vi "get_settings_cluster.vi"(8 "error in (no error)":errorcluster, 11 "GenericPlugin in":refnum<class "StimulatorDL090503.lvclass">) -> (0 "error out":errorcluster, 2 "settings cluster":variant, 3 "GenericPlugin out":refnum<class "StimulatorDL090503.lvclass">)   [LabVIEW 2010, in "StimulatorDL090503.lvclass"]
uses:
  StimulatorDL090503.lvclass
  StimulatorDL090503.lvclass/StimulatorDL090503.ctl
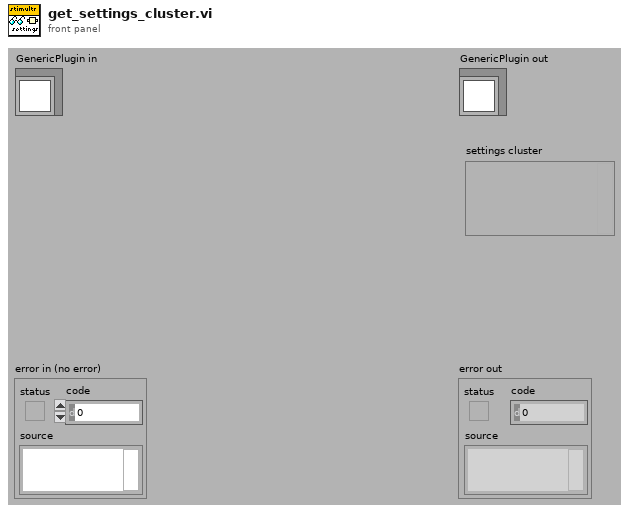
[diagram p1: front panel]
types:
  T1 = typedef "StimulatorDL090503.lvclass/settings_cluster.ctl" = cluster{"application parameters":T2, "pattern":T3}
  T2 = typedef "StimulatorDL090503Scaffold.lvclass/stimulus_application_parameters_cluster.ctl" = cluster{"duration":dbl[unit], "offset":dbl[unit], "repetition period":dbl[unit], "repetitions":i32}
  T3 = typedef "StimulatorDL090503.lvclass/pattern_parameters_cluster.ctl" = cluster{"pattern":T4, "frequency":dbl[unit], "amplitude":dbl, "offset":dbl}
  T4 = typedef "StimulatorDL090503.lvclass/pattern_type_enum.ctl" = enum16{"sine", "square (+/-)", "square (+)", "square (-)"}
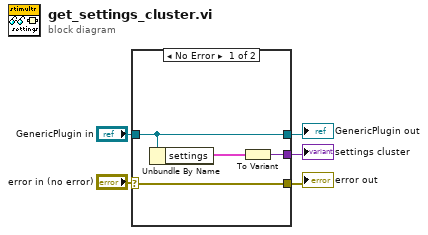
[diagram p0: block diagram]
diagram:
  n1 = case shown="No Error" "error in (no error)" {
    selector: "error in (no error)" -> [w7 w10]
    tunnel: "GenericPlugin in" -> [w6 w11]
    tunnel: [w8 _] -> w4
    tunnel: [w7 w10] -> w2
    tunnel: [w6 w11] -> w1
    frame No Error {
      n2 = Unbundle By Name(w6) -> ("settings"=w9:T1)
      n3 = To Variant(anything=w9) -> (Variant=w8:variant)
    }
    frame Error {
    }
  }
  "error out" <- w2
  "GenericPlugin out" <- w1
  "settings cluster" <- w4
